vi "MultiplexerSendDataIn.vi"(6 "DataIn":bool[](array[boolean]), 7 "Invert":bool, 8 "error in":errorcluster, 9 "RisingEdge":bool, 10 "Clock delay":u32, 11 "Refnum in":T1) -> (0 "error out":errorcluster, 3 "Refnum out":T1)   [LabVIEW 2016]
uses:
  controls/FPGAVIreferenceTypeDef.ctl
  <vilib>/Utility/error.llb/Error Cluster From Error Code.vi
  <vilib>/rvi/errors/niLvFpgaAdjustHostInterfaceError.vi
  <vilib>/rvi/interface/nirviReadWriteControl/nirviReadWriteControl.xnode
  FPGA Bitfiles/qnmController797_usbRIO_controllerFPGAmu.lvbitx
  NiFpgaLv.dll
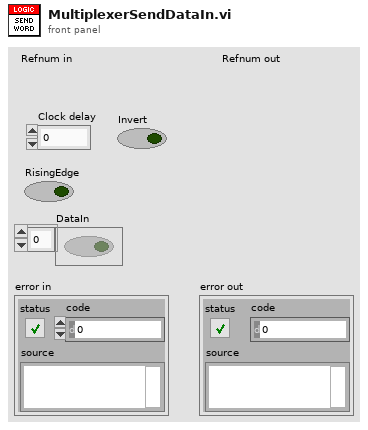
[diagram p1: front panel]
types:
  T1 = typedef "FPGAVIreferenceTypeDef.ctl" = refnum<k20>
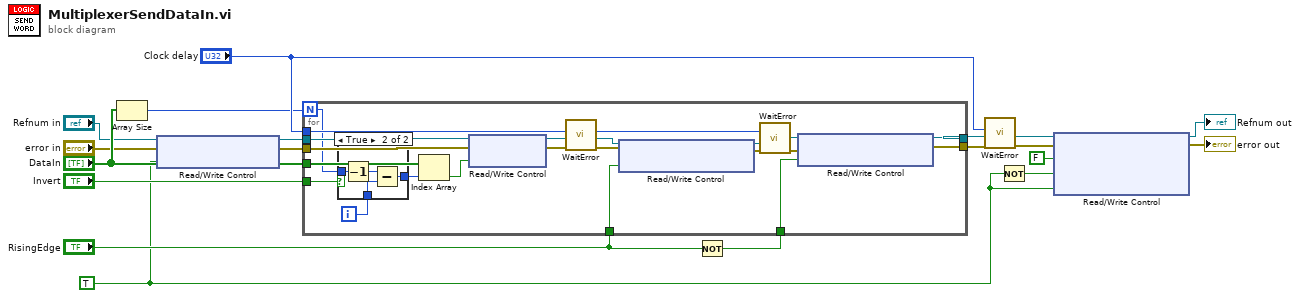
[diagram p0: block diagram]
diagram:
  w1 = TRUE ("dio.p.multiplexerOE")
  n1 = Array Size(array="DataIn") -> (size(s)=w15:i32)
  n2 = xnode "Read/Write Control"("FPGA VI Reference In"="Refnum in", "error in"="error in", "dio.p.multiplexerOE"=w1) -> ("FPGA VI Reference Out"=w9:T1, "error out"=w7:errorcluster)
  n3 = Not(x="RisingEdge") -> (.not. x?=w3:bool)
  n4 = for {
    N: w15 -> [w26]
    tunnel: "Clock delay" -> [w31]
    tunnel: w9 -> [w30]
    tunnel: "DataIn" -> [w27]
    tunnel: "RisingEdge" -> [w29]
    tunnel: w7 -> [w28]
    tunnel: [w24] -> w12
    tunnel: w3 -> [w23]
    tunnel: [w22] -> w11
    tunnel: "Invert" -> [w19]
    i -> [w25]
    n5 = case shown="True" w19 {
      tunnel: w26 -> [_ w42]
      tunnel: w25 -> [w38 w41]
      tunnel: [w38 w40] -> w20
      frame False {
      }
      frame True {
        n6 = Decrement(x=w42) -> (x-1=w39:i32)
        n7 = Subtract(x=w39, y=w41) -> (x-y=w40:i32)
      }
    }
    n8 = Index Array(array=w27, index=w20) -> (element=w21:bool)
    n9 = xnode "Read/Write Control"("FPGA VI Reference In"=w30, "error in"=w28, "dio.i.dataIn"=w21) -> ("FPGA VI Reference Out"=w32:T1, "error out"=w37:errorcluster)
    n10 = call "WaitError.vi"("error in (no error)"=w37, "milliseconds to wait"=w31) -> ("error out"=w36:errorcluster)  [unwired: 9 in]
    n11 = xnode "Read/Write Control"("FPGA VI Reference In"=w32, "error in"=w36, "dio.p.multiplexerclock"=w29) -> ("FPGA VI Reference Out"=w33:T1, "error out"=w35:errorcluster)
    n12 = call "WaitError.vi"("error in (no error)"=w35, "milliseconds to wait"=w31) -> ("error out"=w34:errorcluster)  [unwired: 9 in]
    n13 = xnode "Read/Write Control"("FPGA VI Reference In"=w33, "error in"=w34, "dio.p.multiplexerclock"=w23) -> ("FPGA VI Reference Out"=w24:T1, "error out"=w22:errorcluster)
  }
  n14 = call "WaitError.vi"("error in (no error)"=w11, "milliseconds to wait"="Clock delay") -> ("error out"=w13:errorcluster)  [unwired: 9 in]
  n15 = Not(x=w1) -> (.not. x?=w5:bool)
  n16 = xnode "Read/Write Control"("FPGA VI Reference In"=w12, "error in"=w13, "dio.p.multiplexerclock"=FALSE, "dio.p.multiplexerOE"=w5, "dio.p.multiplexerOE"=w1) -> ("FPGA VI Reference Out"=→"Refnum out":T1, "error out"=→"error out":errorcluster)
